vi "niRFUtil WFM Average (real array).vi"(0 "Data In":T2 min=0 max=127 format="%.2f", 5 "Average Mode":enum16{"Exponential", "Repeat"}(ring), 7 "Average Method":T1, 12 "Reset?":bool=TRUE, 13 "Initialize?":bool=TRUE) -> (4 "Average Data Out":T2 min=0 max=127 format="%.2f")   [LabVIEW 2015, in "niRFUtil.lvlib"]
doc: "(c) Copyright 2006, National Instruments, Inc. This VI may not be duplicated, sold, or distributed without written consent from National Instruments."
uses:
  niRFUtil.lvlib
  Includes/niRFUtil INC Real Array.ctl
  Includes/niRFUtil INC Average Methods.ctl
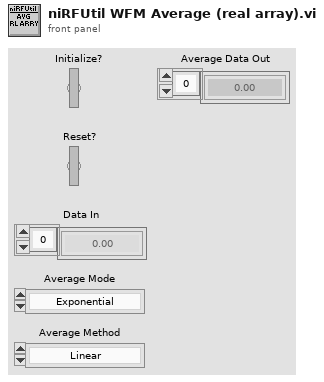
[diagram p1: front panel]
types:
  T1 = typedef "niRFUtil.lvlib/niRFUtil INC Average Methods.ctl" = enum16{"Linear", "Log", "Root", "Max", "Min", "MinMax"}
  T2 = typedef "niRFUtil.lvlib/niRFUtil INC Real Array.ctl" = sgl[]
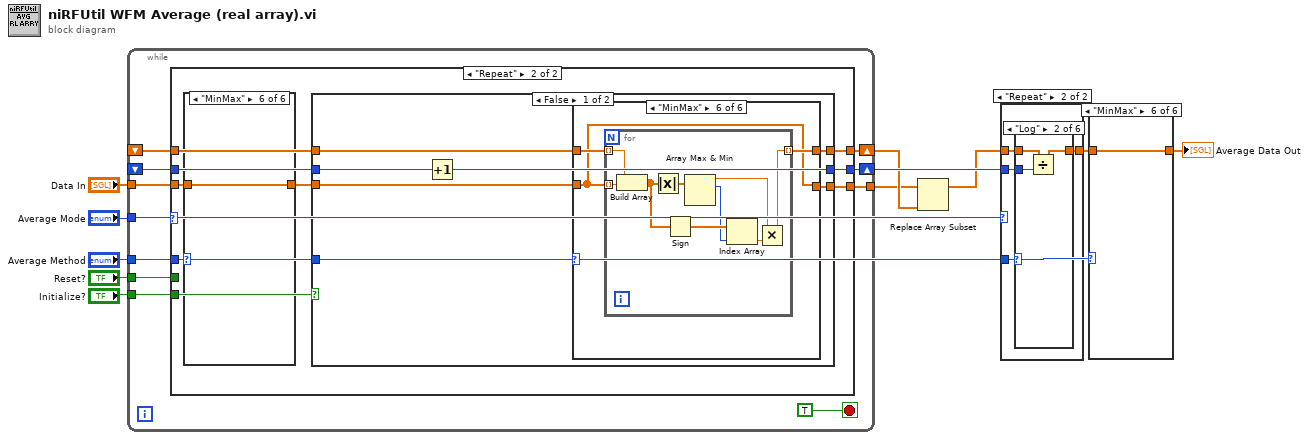
[diagram p0: block diagram]
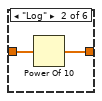
[diagram p3: hidden frame]
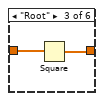
[diagram p4: hidden frame]
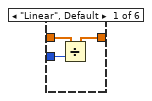
[diagram p8: hidden frame]
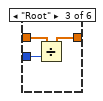
[diagram p9: hidden frame]
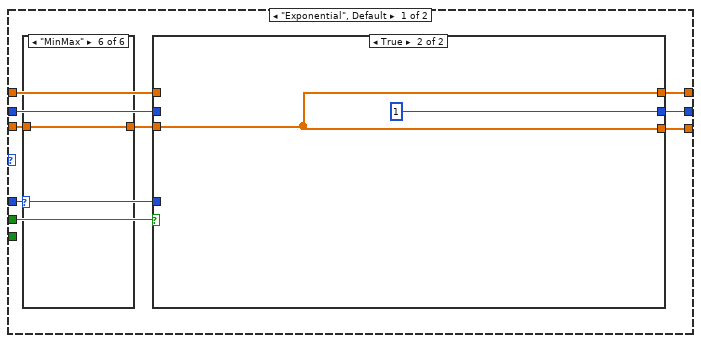
[diagram p13: hidden frame]
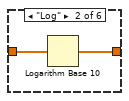
[diagram p15: hidden frame]
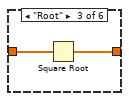
[diagram p16: hidden frame]
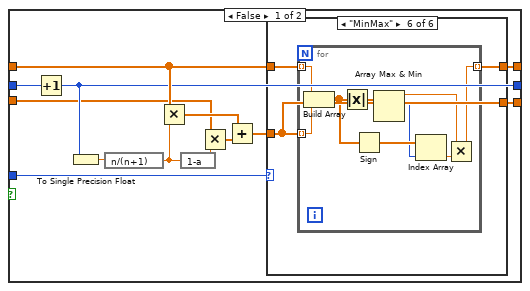
[diagram p19: hidden frame]
diagram:
  n1 = while {
    shift-right: [w19] -> w2
    shift-left: _ -> [w16]
    tunnel: "Average Mode" -> [w21]
    tunnel: "Reset?" -> [w20]
    tunnel: "Data In" -> [w18]
    shift-right: [w17] -> w11
    shift-left: _ -> [w15]
    tunnel: "Average Method" -> [w14]
    tunnel: "Initialize?" -> [w13]
    tunnel: [w12] -> w1
    stop <- TRUE stop-if-true
    n2 = case shown="\"Repeat\"" w21 {
      tunnel: w20 -> [w28 _]
      tunnel: [w31 w84] -> w19
      tunnel: w18 -> [w26 w79]
      tunnel: [w27 w81] -> w17
      tunnel: w16 -> [w30 w83]
      tunnel: w15 -> [w29 w82]
      tunnel: w14 -> [w24 w77]
      tunnel: w13 -> [_ w80]
      tunnel: [w23 w76] -> w12
      frame "Exponential", Default {
        n3 = case shown="\"MinMax\"" w24 {
          tunnel: w26 -> [w32 w34 w36 w37 w38 w39]
          tunnel: [w32 w33 w35 w37 w38 w39] -> w25
          frame "Linear", Default {
          }
          frame "Log" {
            n4 = Logarithm Base 10(1:w34) -> (0:w33:T2)
          }
          frame "Root" {
            n5 = Square Root(x=w36) -> (sqrt(x)=w35:T2)
          }
          frame "Max" {
          }
          frame "Min" {
          }
          frame "MinMax" {
          }
        }
        n6 = case shown="True" w28 {
          tunnel: w25 -> [w41 w74]
          tunnel: [w47 w74] -> w31
          tunnel: w30 -> [w45 _]
          tunnel: w29 -> [w44 _]
          tunnel: [w43 1] -> w27
          tunnel: w24 -> [w42 _]
          tunnel: [w40 w74] -> w23
          frame False {
            n7 = Increment(x=w44) -> (x+1=w43:i32)
            n8 = To Single Precision Float(number=w43) -> (single precision float=w52:sgl)
            n9 = expression code="n/(n+1)"(w52) -> (w51:sgl)
            n10 = Multiply(x=w45, y=w51) -> (x*y=w48:T2)
            n11 = expression code="1-a"(w51) -> (w50:sgl)
            n12 = Multiply(x=w41, y=w50) -> (x*y=w49:T2)
            n13 = Add(x=w48, y=w49) -> (x+y=w46:T2)
            n14 = case shown="\"MinMax\"" w42 {
              tunnel: [w53 w54 w55 w57 w60 w63] -> w47
              tunnel: w46 -> [w53 w54 w55 w56 w59 w62]
              tunnel: w45 -> [_ _ _ w58 w61 w64]
              tunnel: [w53 w54 w55 w56 w59 w62] -> w40
              frame "Linear", Default {
              }
              frame "Log" {
              }
              frame "Root" {
              }
              frame "Max" {
                n15 = Max & Min(x=w58, y=w56) -> (max(x,y)=w57:T2)  [unwired: 1 out]
              }
              frame "Min" {
                n16 = Max & Min(x=w61, y=w59) -> (min(x,y)=w60:T2)  [unwired: 1 out]
              }
              frame "MinMax" {
                n17 = for {
                  tunnel: w64 -> [w70] mode=indexing
                  tunnel: w62 -> [w69] mode=indexing
                  tunnel: [w68] -> w63 mode=indexing
                  n18 = Build Array(w70, w69) -> (w73:sgl[])
                  n19 = Absolute Value(x=w73) -> (abs(x)=w67:sgl[])
                  n20 = Sign(1:w73) -> (0:w72:sgl[])
                  n21 = Array Max & Min(array=w67) -> (max value=w66:sgl, max index (indices)=w65:i32)  [unwired: 2 out]
                  n22 = Index Array(array=w72, index=w65) -> (element=w71:sgl)
                  n23 = Multiply(x=w66, y=w71) -> (x*y=w68:sgl)
                }
              }
            }
          }
          frame True {
          }
        }
      }
      frame "Repeat" {
        n24 = case shown="\"MinMax\"" w77 {
          tunnel: w79 -> [w85 w87 w89 w90 w91 w92]
          tunnel: [w85 w86 w88 w90 w91 w92] -> w78
          frame "Linear", Default {
          }
          frame "Log" {
            n25 = Logarithm Base 10(1:w87) -> (0:w86:T2)
          }
          frame "Root" {
            n26 = Square Root(x=w89) -> (sqrt(x)=w88:T2)
          }
          frame "Max" {
          }
          frame "Min" {
          }
          frame "MinMax" {
          }
        }
        n27 = case shown="False" w80 {
          tunnel: w78 -> [w93 w127]
          tunnel: [w99 w127] -> w84
          tunnel: w83 -> [w98 _]
          tunnel: w82 -> [w97 _]
          tunnel: [w96 1] -> w81
          tunnel: w77 -> [w95 _]
          tunnel: [w94 w127] -> w76
          frame False {
            n28 = Increment(x=w97) -> (x+1=w96:i32)
            n29 = case shown="\"MinMax\"" w95 {
              tunnel: [w101 w104 w107 w110 w113 w116] -> w99
              tunnel: w98 -> [w102 w105 w108 w111 w114 w117]
              tunnel: w93 -> [w100 w103 w106 w109 w112 w115]
              tunnel: [w100 w103 w106 w109 w112 w115] -> w94
              frame "Linear", Default {
                n30 = Add(x=w102, y=w100) -> (x+y=w101:T2)
              }
              frame "Log" {
                n31 = Add(x=w105, y=w103) -> (x+y=w104:T2)
              }
              frame "Root" {
                n32 = Add(x=w108, y=w106) -> (x+y=w107:T2)
              }
              frame "Max" {
                n33 = Max & Min(x=w111, y=w109) -> (max(x,y)=w110:T2)  [unwired: 1 out]
              }
              frame "Min" {
                n34 = Max & Min(x=w114, y=w112) -> (min(x,y)=w113:T2)  [unwired: 1 out]
              }
              frame "MinMax" {
                n35 = for {
                  tunnel: w117 -> [w123] mode=indexing
                  tunnel: [w122] -> w116 mode=indexing
                  tunnel: w115 -> [w120] mode=indexing
                  n36 = Build Array(w123, w120) -> (w126:sgl[])
                  n37 = Absolute Value(x=w126) -> (abs(x)=w121:sgl[])
                  n38 = Sign(1:w126) -> (0:w125:sgl[])
                  n39 = Array Max & Min(array=w121) -> (max value=w118:sgl, max index (indices)=w119:i32)  [unwired: 2 out]
                  n40 = Index Array(array=w125, index=w119) -> (element=w124:sgl)
                  n41 = Multiply(x=w118, y=w124) -> (x*y=w122:sgl)
                }
              }
            }
          }
          frame True {
          }
        }
      }
    }
  }
  n42 = Replace Array Subset(array=w1, new element=w2) -> (w3:T2)  [unwired: 1 in]
  n43 = case shown="\"Repeat\"" "Average Mode" {
    tunnel: [w129 w131] -> w5
    tunnel: w3 -> [w129 w132]
    tunnel: w11 -> [_ w133]
    tunnel: "Average Method" -> [_ w130]
    frame "Exponential", Default {
    }
    frame "Repeat" {
      n44 = case shown="\"Log\"" w130 {
        tunnel: w133 -> [w136 w139 w142 _ _ _]
        tunnel: w132 -> [w135 w138 w141 w143 w144 w145]
        tunnel: [w134 w137 w140 w143 w144 w145] -> w131
        frame "Linear", Default {
          n45 = Divide(x=w135, y=w136) -> (x/y=w134:T2)
        }
        frame "Log" {
          n46 = Divide(x=w138, y=w139) -> (x/y=w137:T2)
        }
        frame "Root" {
          n47 = Divide(x=w141, y=w142) -> (x/y=w140:T2)
        }
        frame "Max" {
        }
        frame "Min" {
        }
        frame "MinMax" {
        }
      }
    }
  }
  n48 = case shown="\"MinMax\"" "Average Method" {
    tunnel: w5 -> [w146 w148 w150 w151 w152 w153]
    tunnel: [w146 w147 w149 w151 w152 w153] -> w4
    frame "Linear", Default {
    }
    frame "Log" {
      n49 = Power Of 10(x=w148) -> (10^x=w147:T2)
    }
    frame "Root" {
      n50 = Square(x=w150) -> (x^2=w149:T2)
    }
    frame "Max" {
    }
    frame "Min" {
    }
    frame "MinMax" {
    }
  }
  "Average Data Out" <- w4
